vi "Test Set Return Value.vi"(8 "error in (no error)":errorcluster, 11 "Test Case In":refnum<class "Return Value Test.lvclass">) -> (0 "error out":errorcluster, 3 "Test Case Out":refnum<class "Return Value Test.lvclass">)   [LabVIEW 2020, in "Return Value Test.lvclass"]
uses:
  Return Value Test.lvclass
  C:/Program Files (x86)/National Instruments/LabVIEW 2020/vi.lib/Astemes/LUnit/Test Case.lvclass
  <vilib>/Astemes/LUnit/Test Case.lvclass/Test Case.ctl
  4993e8ee-a06a-463a-9684-69129f64d5ce.vi
  <vilib>/Astemes/LUnit/Append Pass Result.vi
  <vilib>/Astemes/LUnit/Append Fail Result.vi
  <vilib>/Astemes/LUnit/Describe Comparison.vi
  <vilib>/Astemes/LUnit/Compare Variants.vi
  <vilib>/Astemes/LUnit/Variant to string.vi
  <vilib>/Utility/Data Type/Get Type Information.vi
  <vilib>/Utility/LVClass/Get LV Class Name.vi
  Test Doubles/Test Interface Responsive Mock/Test Interface Responsive Mock.lvclass
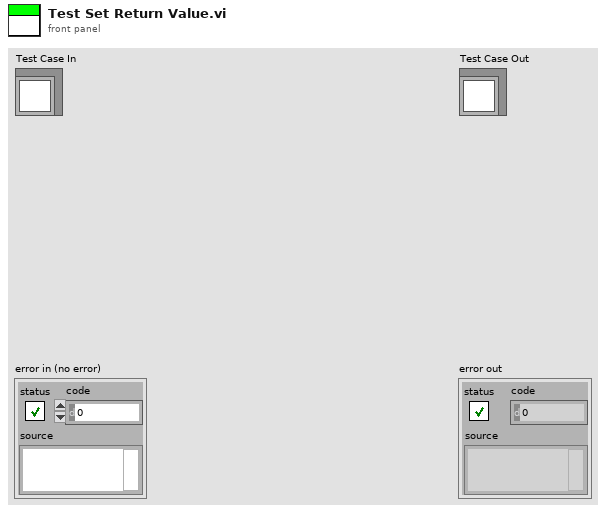
[diagram p1: front panel]
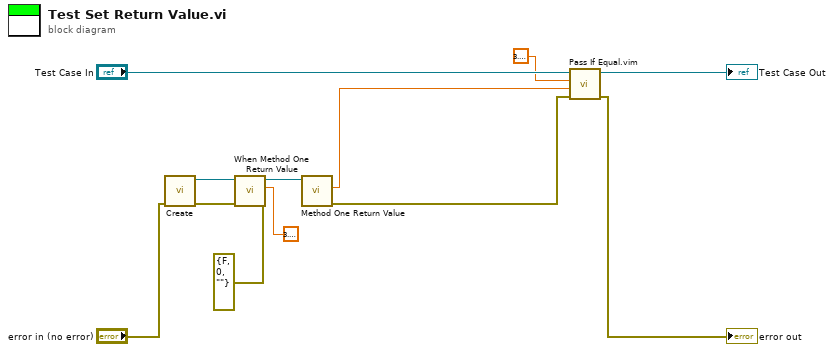
[diagram p0: block diagram]
diagram:
  n1 = call "Create.vi"("error in (no error)"="error in (no error)") -> ("error out"=w8:errorcluster, "Test Interface Mock Out"=w9:refnum<class "Test Interface Responsive Mock.lvclass">)  [unwired: 9 in]
  n2 = call "When Method One Return Value.vi"("error out"=errorcluster {"status"=FALSE, "code"=0, "source"=""}, "Return Value"=3.141592653589793, "error in (no error)"=w8, "Test Interface Mock In"=w9) -> ("Test Interface Mock Out"=w7:refnum<class "Test Interface Responsive Mock.lvclass">)  [unwired: 7 in]
  n3 = call-dynamic "Method One Return Value.vi"("Test Interface Mock in"=w7) -> ("error out"=w3:errorcluster, "Return Value"=w5:dbl)  [unwired: 8 in, 1 out]
  n4 = call "Pass If Equal.vim"("error in (no error)"=w3, "Actual"=w5, "Expected"=3.141592653589793, "LUnit Test Case In"="Test Case In") -> ("error out"=→"error out":errorcluster, "LUnit Test Case Out"=→"Test Case Out":refnum<class "Return Value Test.lvclass">)  [unwired: 6 in]
